vi "CUMain.vi"() -> ()   [LabVIEW 2013]
doc: "Use this template to build a simple state machine design pattern. Each state executes code and determines which state to transition to."
uses:
  controls/CUState.ctl
  controls/CUData.ctl
  <vilib>/Instr/_visa.llb/VISA Configure Serial Port (Instr).vi
panel:
  in  "Disable Encode":bool
  out "Data content":string
  out "Data length":string
  out "Package describer":string
  out "Counter":string
  in  "Send A-V command":bool
  in  "Value (U16)":u16 format="%04x"
  in  "Address (U16)":u16=255 format="%04x"
  in  "Keep send encode string":bool
  in  "Enable read":bool=TRUE
  out "Raw string":string
  in  "Bytes to read":u32=512
  out "Actual bytes read":u32
  in  "Clear text":bool
  out "Encoded string":string
  in  "Send string":string="DA1 0C1 <<< SM1 SM2 SM3 >>> MM1"
  in  "data bits":u16=8 min=5 max=8 step=1
  in  "VISA resource name":refnum<visa-resource-name>="COM1"
  in  "baud rate":u32=9600
  in  "Stop Button":bool
  in  "Send ASCII command":bool
  # "CU Console"
  # "(Add SPACE between ASCII commands)"
  # "(Press ENTER to send when value ready)"
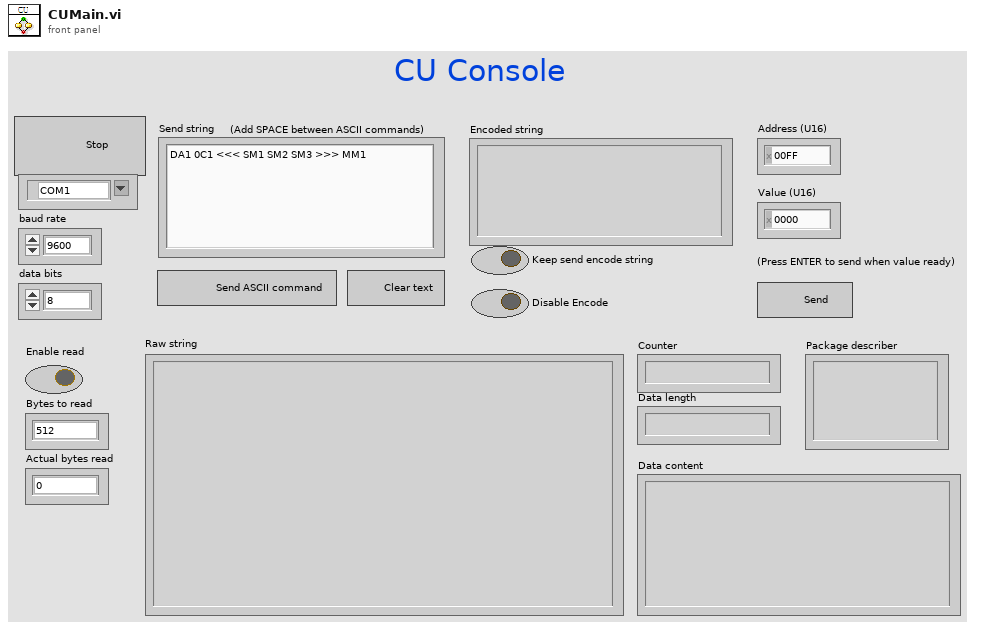
[diagram p1: front panel]
types:
  T1 = typedef "CUData.ctl" = cluster{"String to send":string, "Encoded string to send":string, "Raw string":string}
  T2 = typedef "CUState.ctl" = enum16{"Initialize", "Wait for Event", "Encode ASCII command", "Encode A-V command", "Send command", "Read data", "Decode Science data", "Stop"}
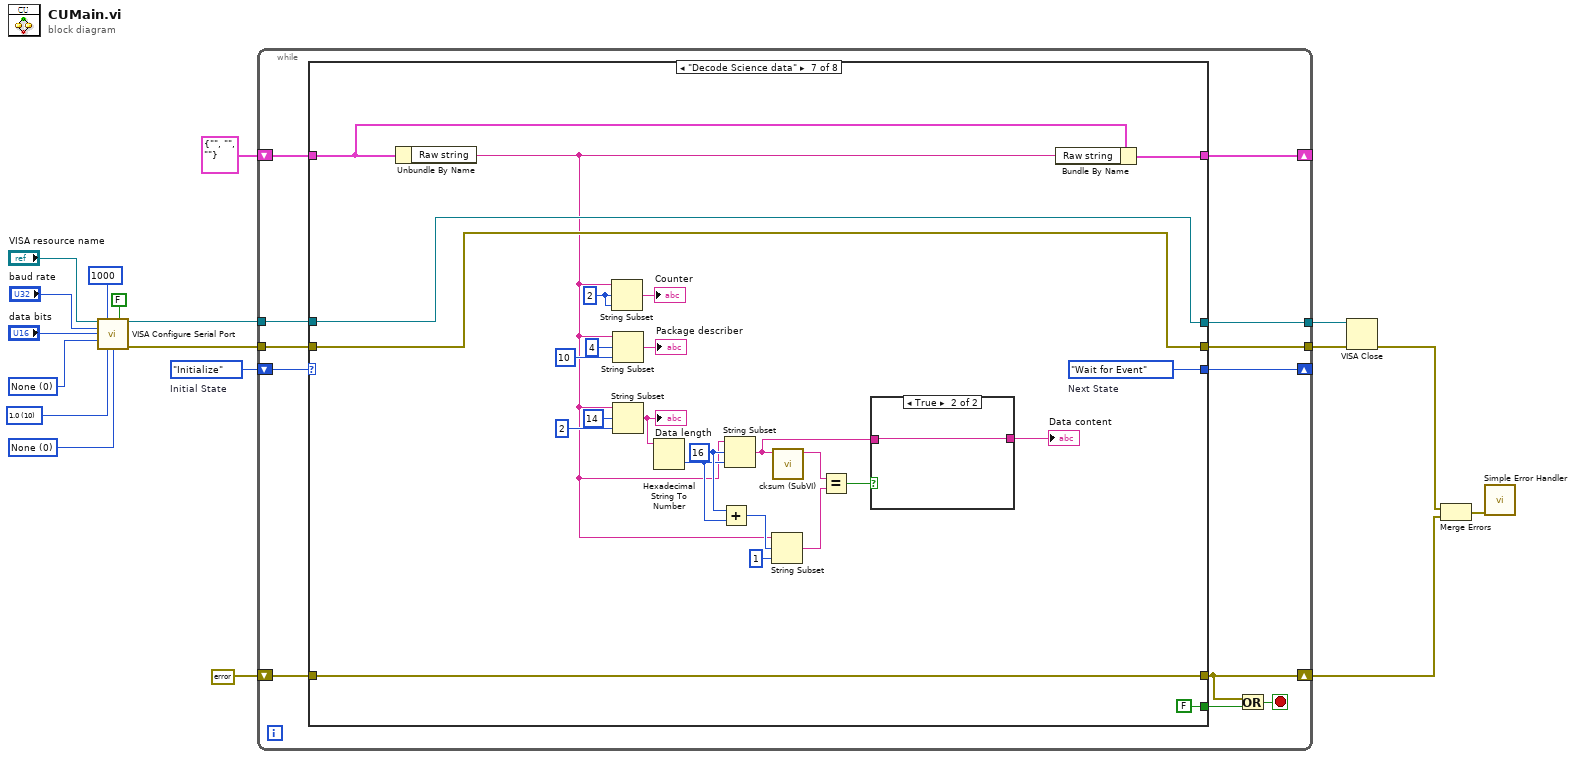
[diagram p0: block diagram]
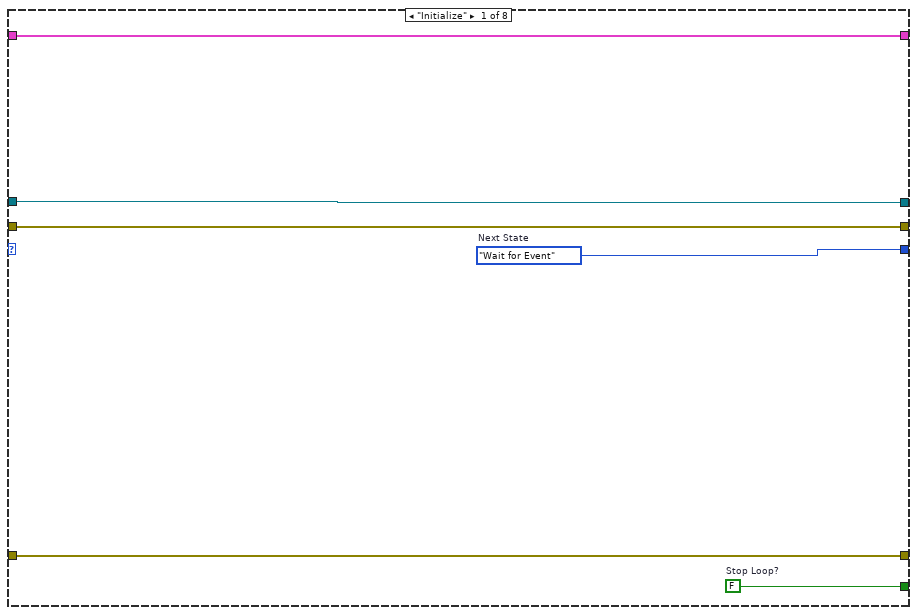
[diagram p2: hidden frame]
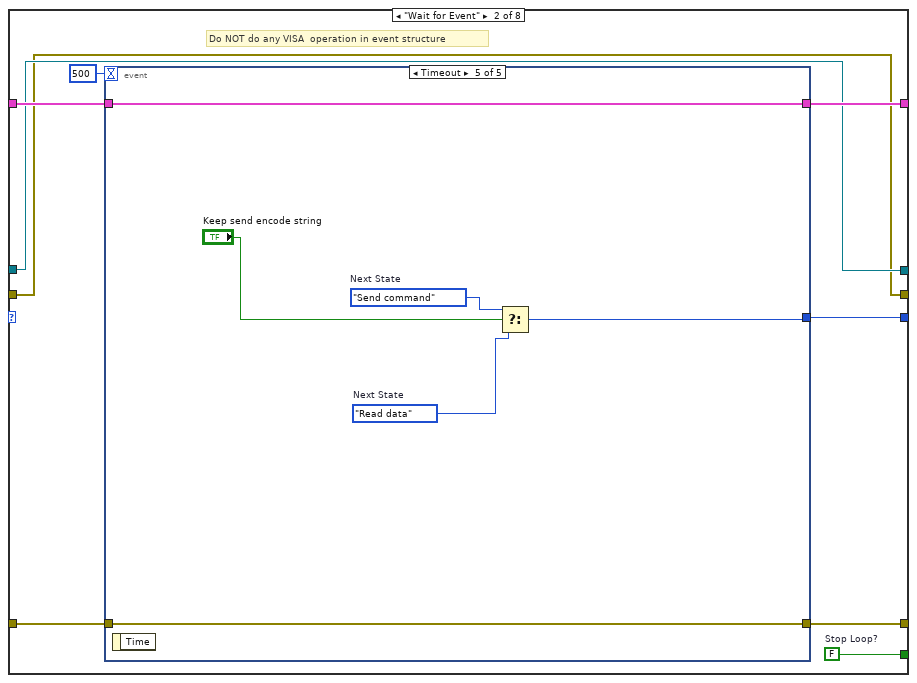
[diagram p3: hidden frame]
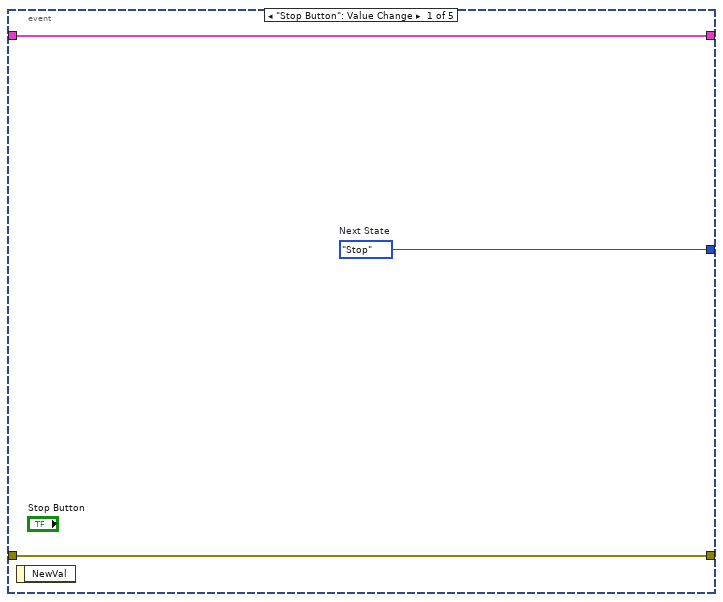
[diagram p4: hidden frame]
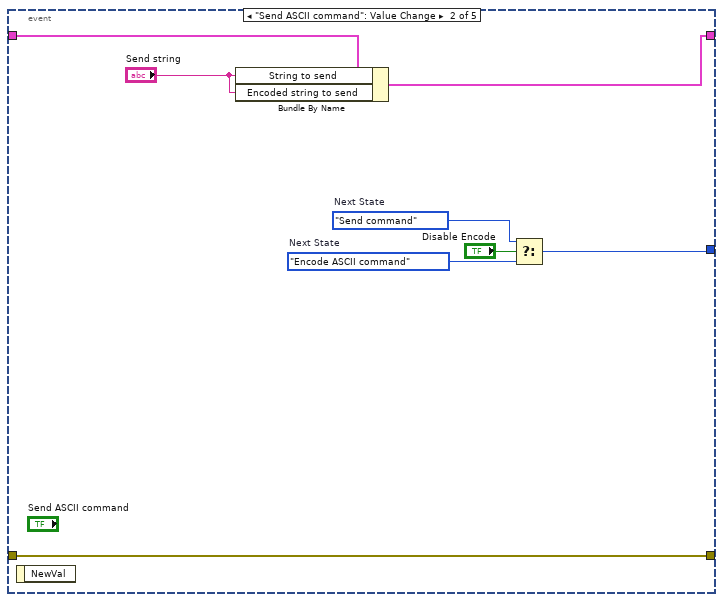
[diagram p5: hidden frame]
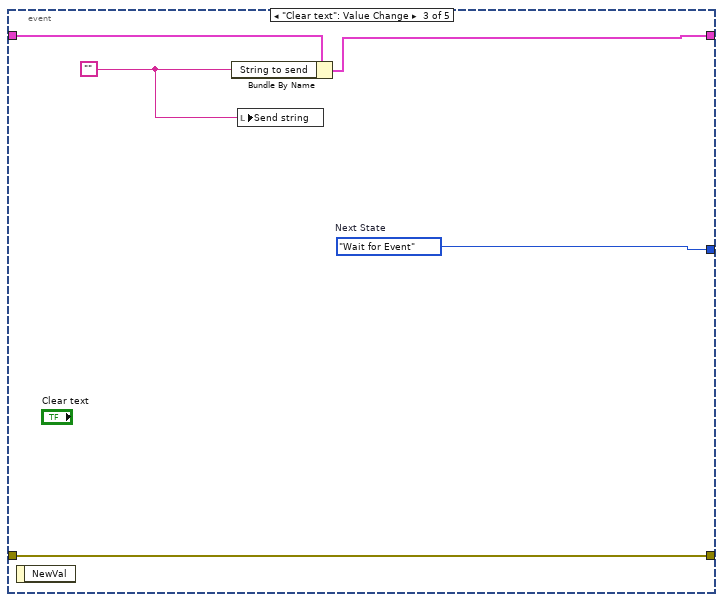
[diagram p6: hidden frame]
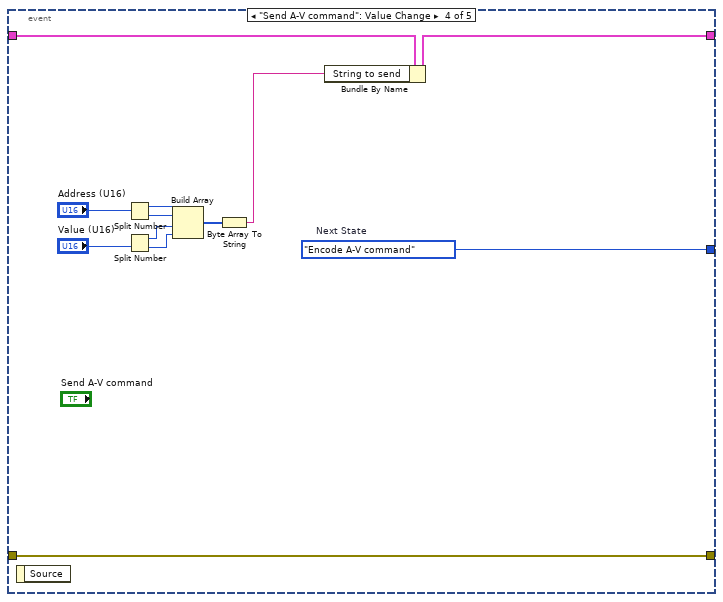
[diagram p7: hidden frame]
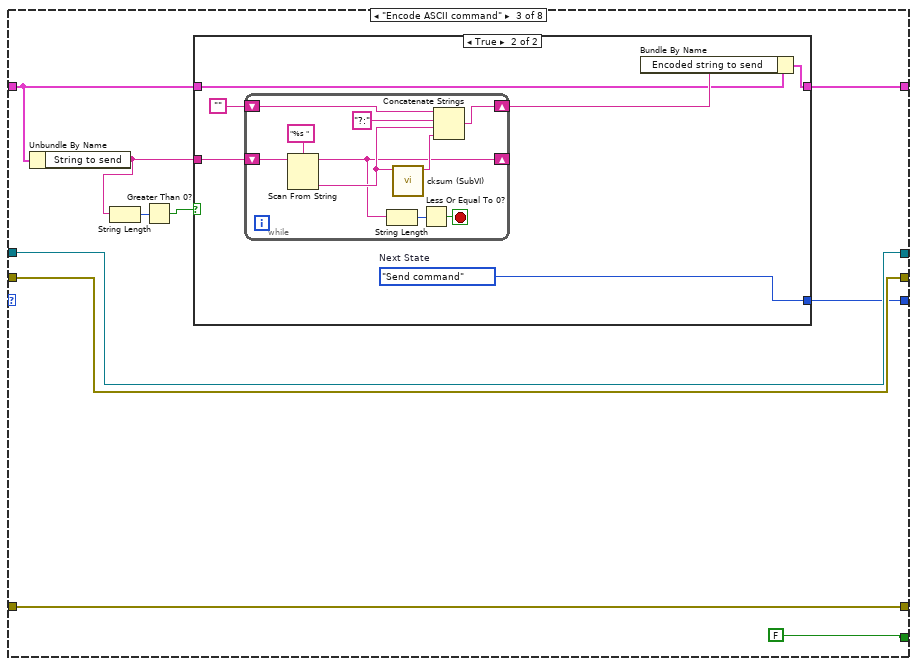
[diagram p8: hidden frame]
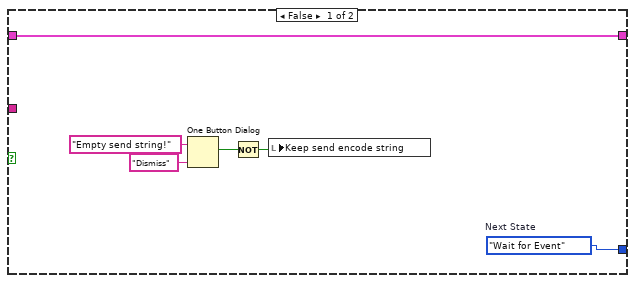
[diagram p9: hidden frame]
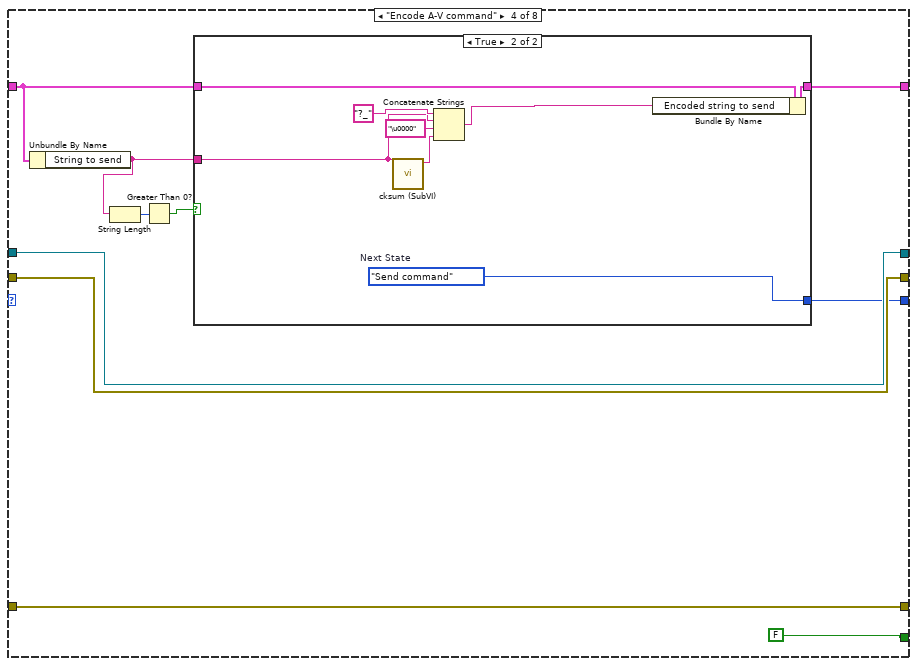
[diagram p10: hidden frame]
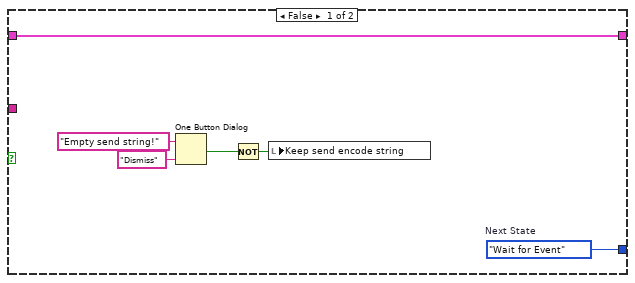
[diagram p11: hidden frame]
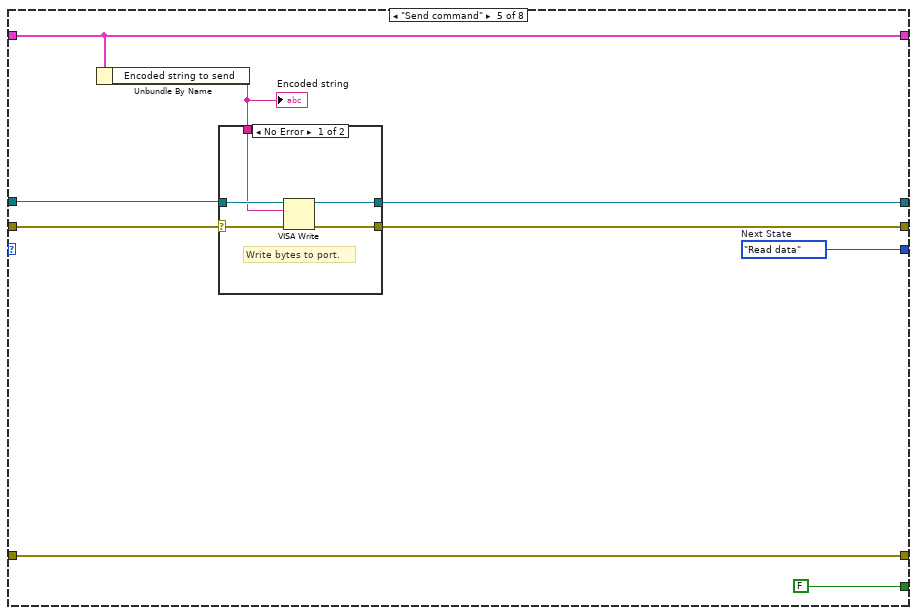
[diagram p12: hidden frame]
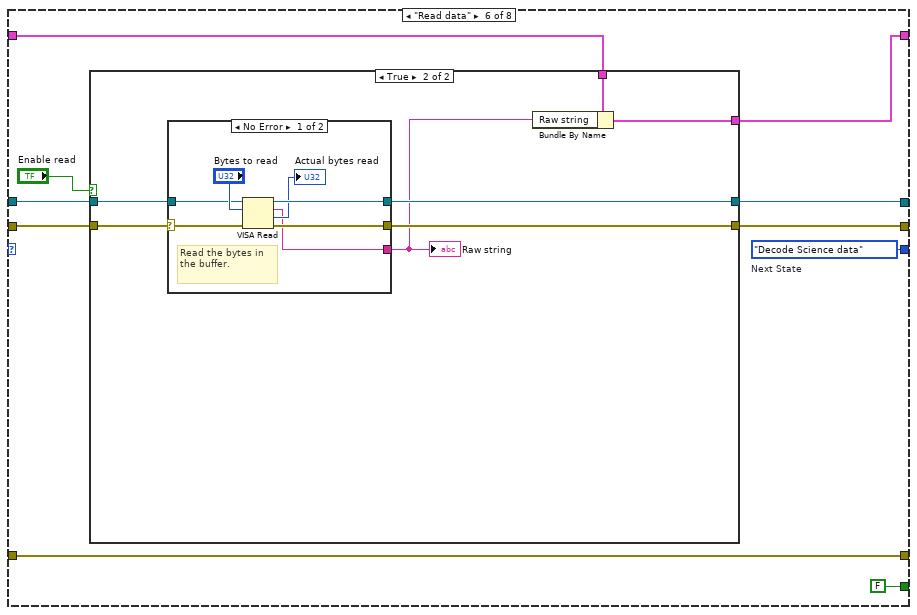
[diagram p14: hidden frame]
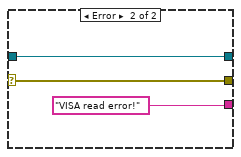
[diagram p16: hidden frame]
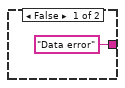
[diagram p17: hidden frame]
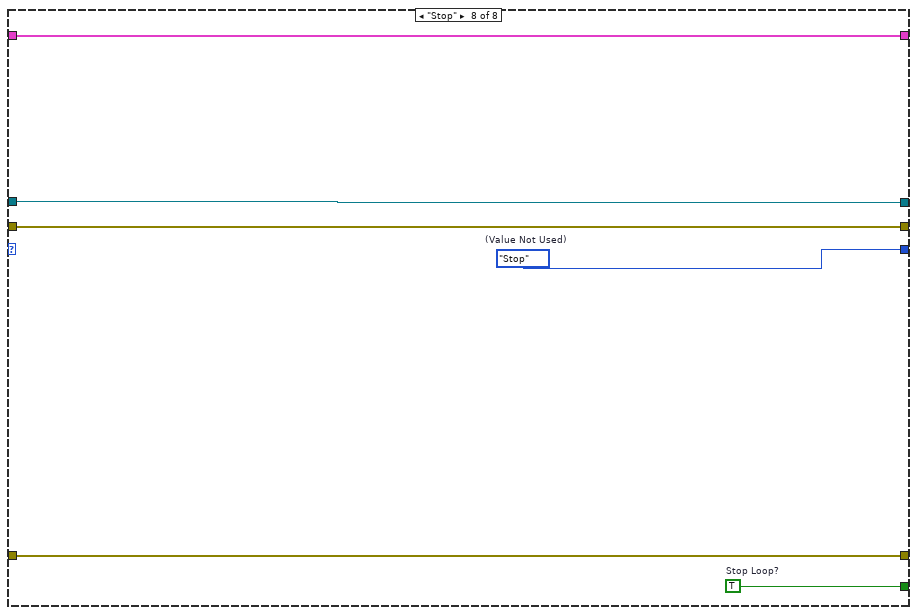
[diagram p18: hidden frame]
diagram:
  w12 = u16 10 items=["1.0"=10, "1.5"=15, "2.0"=20] ("stop bits")
  w13 = u16 0 items=["None", "Odd", "Even", "Mark", "Space"] ("parity")
  w9 = u16 0 items=["None"=0, "XON/XOFF"=1, "RTS/CTS"=2, "DTR/DSR"=4] ("flow control")
  w18 = CUState."Initialize"  # Initial State
  n1 = call-poly "VISA Configure Serial Port"("VISA resource name"="VISA resource name", "timeout (10sec)"=u32 1000 ("timeout (ms)"), "Enable Termination\nChar (T)"=FALSE ("End read on termination character?"), "baud rate (9600)"="baud rate", "data bits (8)"="data bits", "parity (0:none)"=w13, "stop bits (10: 1 bit)"=w12, "flow control (0:none)"=w9) -> ("VISA resource name out"=w6:refnum<visa-resource-name>, "error out"=w5:errorcluster)  [unwired: 2 in, 4 out]
  n2 = while {
    shift-right: [w29] -> _
    shift-left: w18 -> [w30]
    shift-right: [w27] -> _
    shift-left: T1 {"String to send"="", "Encoded string to send"="", "Raw string"=""} ("Data") -> [w28]
    shift-right: [w23] -> w1
    shift-left: errorcluster {"status"=FALSE, "code"=0, "source"=""} ("error constant") -> [w26]
    tunnel: [w22] -> w7
    tunnel: w6 -> [w21]
    tunnel: w5 -> [w20]
    tunnel: [w19] -> w4
    stop <- w24 stop-if-true
    n3 = case shown="\"Decode Science data\"" w30 {
      tunnel: [w36 w45 w86 w118 w144 w154 w187 w214] -> w29
      tunnel: [w35 w44 FALSE ("Stop Loop?") FALSE ("Stop Loop?") FALSE ("Stop Loop?") FALSE ("Stop Loop?") FALSE ("Stop Loop?") w212] -> w25
      tunnel: w28 -> [w31 w43 w84 w116 w136 w153 w184 w213]
      tunnel: [w31 w42 w83 w115 w136 w152 w185 w213] -> w27
      tunnel: w26 -> [w34 w41 w89 w121 w142 w161 w206 w211]
      tunnel: [w34 w40 w89 w121 w142 w161 w206 w211] -> w23
      tunnel: [w33 w39 w88 w120 w140 w159 w189 w210] -> w22
      tunnel: w21 -> [w33 w39 w88 w120 w141 w160 w189 w210]
      tunnel: w20 -> [w32 w38 w87 w119 w138 w157 w188 w209]
      tunnel: [w32 w38 w87 w119 w139 w158 w188 w209] -> w19
      frame "Initialize" {
        w35 = FALSE  # Stop Loop?
        w36 = CUState."Wait for Event"  # Next State
      }
      frame "Wait for Event" {
        w44 = FALSE  # Stop Loop?
        # "Do NOT do any VISA  operation in event structure"
        n4 = event shown="[4] Timeout" {
          selector: _ -> [_ _ _ _ _]
          dyn-events: _ -> [_ _ _ _ _]
          timeout: 500 -> [_ _ _ _ _]
          tunnel: [w48 w53 w58 w73 w76] -> w45
          tunnel: w43 -> [w47 w56 w60 w72 w78]
          tunnel: [w47 w55 w59 w71 w78] -> w42
          tunnel: w41 -> [w46 w54 w61 w70 w79]
          tunnel: [w46 w54 w61 w70 w79] -> w40
          event "Stop Button": Value Change {
            w48 = CUState."Stop"  # Next State
            n5 = event-data() -> ()  [unwired: 1 in, 1 out]
          }
          event "Send ASCII command": Value Change {
            w51 = CUState."Send command"  # Next State
            w52 = CUState."Encode ASCII command"  # Next State
            n6 = event-data() -> ()  [unwired: 1 in, 1 out]
            n7 = Bundle By Name(cluster=w56, "String to send"="Send string", "Encoded string to send"="Send string") -> (w55:T1)
            n8 = Select(t=w51, s="Disable Encode", f=w52) -> (s? t:f=w53:T2)
          }
          event "Clear text": Value Change {
            w58 = CUState."Wait for Event"  # Next State
            w57 = "" ("String to send")
            n9 = event-data() -> ()  [unwired: 1 in, 1 out]
            n10 = Bundle By Name(cluster=w60, "String to send"=w57) -> (w59:T1)
            n11 = local write "Send string"(w57) -> ()
          }
          event "Send A-V command": Value Change {
            w73 = CUState."Encode A-V command"  # Next State
            n12 = event-data() -> ()  [unwired: 1 in, 1 out]
            n13 = Split Number(x="Address (U16)") -> (hi(x)=w67:u8, lo(x)=w66:u8)
            n14 = Split Number(x="Value (U16)") -> (hi(x)=w65:u8, lo(x)=w64:u8)
            n15 = Build Array(w67, w66, w65, w64) -> (w63:u8[])
            n16 = Byte Array To String(unsigned byte array=w63) -> (string=w62:string)
            n17 = Bundle By Name(cluster=w72, "String to send"=w62) -> (w71:T1)
          }
          event Timeout {
            w75 = CUState."Send command"  # Next State
            w74 = CUState."Read data"  # Next State
            n18 = event-data() -> ()  [unwired: 1 in, 1 out]
            n19 = Select(t=w75, s="Keep send encode string", f=w74) -> (s? t:f=w76:T2)
          }
        }
      }
      frame "Encode ASCII command" {
        n20 = Unbundle By Name(w84) -> ("String to send"=w81:string)
        n21 = String Length(string=w81) -> (length=w82:i32)
        n22 = Greater Than 0?(x=w82) -> (x > 0?=w80:bool)
        n23 = case shown="True" w80 {
          tunnel: [w95 w101] -> w86
          tunnel: w81 -> [_ w100]
          tunnel: w84 -> [w93 w98]
          tunnel: [w93 w97] -> w83
          frame False {
            w95 = CUState."Wait for Event"  # Next State
            n24 = One Button Dialog(message="Empty send string!", button name ("OK")="Dismiss") -> (true=w90:bool)
            n25 = Not(x=w90) -> (.not. x?=w91:bool)
            n26 = local write "Keep send encode string"(w91) -> ()
          }
          frame True {
            w101 = CUState."Send command"  # Next State
            n27 = while {
              shift-right: [w104] -> _
              shift-left: w100 -> [w111]
              shift-right: [w107] -> w99
              shift-left: "" -> [w102]
              stop <- w108 stop-if-true
              n28 = Scan From String(format string="%s ", input string=w111) -> (remaining string=w104:string, output 1=w106:string)  [unwired: 3 in, 2 out]
              n29 = String Length(string=w104) -> (length=w109:i32)
              n30 = call "cksum (SubVI).vi"("Input String"=w106) -> ("Checksum"=w105:string)  [unwired: 10 in]
              n31 = Less Or Equal To 0?(x=w109) -> (x <= 0?=w108:bool)
              n32 = Concatenate Strings(w102, "?:", w106, w105) -> (w107:string)
            }
            n33 = Bundle By Name(cluster=w98, "Encoded string to send"=w99) -> (w97:T1)
          }
        }
      }
      frame "Encode A-V command" {
        n34 = Unbundle By Name(w116) -> ("String to send"=w113:string)
        n35 = String Length(string=w113) -> (length=w114:i32)
        n36 = Greater Than 0?(x=w114) -> (x > 0?=w112:bool)
        n37 = case shown="True" w112 {
          tunnel: [w127 w135] -> w118
          tunnel: w113 -> [_ w129]
          tunnel: w116 -> [w125 w133]
          tunnel: [w125 w132] -> w115
          frame False {
            w127 = CUState."Wait for Event"  # Next State
            n38 = One Button Dialog(message="Empty send string!", button name ("OK")="Dismiss") -> (true=w122:bool)
            n39 = Not(x=w122) -> (.not. x?=w123:bool)
            n40 = local write "Keep send encode string"(w123) -> ()
          }
          frame True {
            w135 = CUState."Send command"  # Next State
            n41 = call "cksum (SubVI).vi"("Input String"=w129) -> ("Checksum"=w131:string)  [unwired: 10 in]
            n42 = Concatenate Strings("?_", w129, "\u0000" ("string"), w131) -> (w134:string)
            n43 = Bundle By Name(cluster=w133, "Encoded string to send"=w134) -> (w132:T1)
          }
        }
      }
      frame "Send command" {
        w144 = CUState."Read data"  # Next State
        n44 = Unbundle By Name(w136) -> ("Encoded string to send"=w137:string)
        "Encoded string" <- w137
        n45 = case shown="No Error" w138 {
          selector: w138 -> [w146 w151]
          tunnel: [w149 w150] -> w140
          tunnel: [w148 w151] -> w139
          tunnel: w141 -> [w147 w150]
          tunnel: w137 -> [w145 _]
          frame No Error {
            # "Write bytes to port."
            n46 = VISA Write(VISA resource name=w147, write buffer=w145, error in (no error)=w146) -> (VISA resource name out=w149:refnum<visa-resource-name>, error out=w148:errorcluster)  [unwired: 1 out]
          }
          frame Error {
          }
        }
      }
      frame "Read data" {
        w154 = CUState."Decode Science data"  # Next State
        n47 = case shown="True" "Enable read" {
          tunnel: w160 -> [w164 w171]
          tunnel: [w164 w170] -> w159
          tunnel: [w163 w169] -> w158
          tunnel: w157 -> [w163 w168]
          tunnel: w153 -> [w162 w167]
          tunnel: [w162 w165] -> w152
          frame False {
          }
          frame True {
            n48 = case "Read bytes from port." shown="No Error" w168 {
              selector: w168 -> [w174 w180]
              tunnel: [w177 w180] -> w169
              tunnel: [w178 w181] -> w170
              tunnel: w171 -> [w175 w181]
              tunnel: [w172 "VISA read error!" ("read buffer")] -> w166
              frame No Error {
                # "Read the bytes in the buffer."
                n49 = VISA Read(VISA resource name=w175, byte count="Bytes to read", error in (no error)=w174) -> (VISA resource name out=w178:refnum<visa-resource-name>, read buffer=w172:string, return count=→"Actual bytes read":u32, error out=w177:errorcluster)
              }
              frame Error {
                # "Error occurred \nreading Bytes at \nSerial Port"
              }
            }
            "Raw string" <- w166
            n50 = Bundle By Name(cluster=w167, "Raw string"=w166) -> (w165:T1)
          }
        }
      }
      frame "Decode Science data" {
        w187 = CUState."Wait for Event"  # Next State
        w197 = u32 16 ("offset (0)")
        w198 = 2 ("offset (0)")
        n51 = Unbundle By Name(w184) -> ("Raw string"=w183:string)
        n52 = String Subset(string=w183, offset (0)=w198, length (rest)=w198) -> (substring=→"Counter":string)
        n53 = String Subset(string=w183, offset (0)=4, length (rest)=10 ("length (rest)")) -> (substring=→"Package describer":string)
        n54 = String Subset(string=w183, offset (0)=14, length (rest)=2 ("length (rest)")) -> (substring=w200:string)
        "Data length" <- w200
        n55 = Hexadecimal String To Number(string=w200) -> (number=w196:u32)  [unwired: 2 in, 1 out]
        n56 = Add(x=w197, y=w196) -> (x+y=w195:u32)
        n57 = String Subset(string=w183, offset (0)=w197, length (rest)=w196) -> (substring=w190:string)
        n58 = String Subset(string=w183, offset (0)=w195, length (rest)=1 ("length (rest)")) -> (substring=w192:string)
        n59 = call "cksum (SubVI).vi"("Input String"=w190) -> ("Checksum"=w193:string)  [unwired: 10 in]
        n60 = Equal?(x=w193, y=w192) -> (x = y?=w191:bool)
        n61 = case shown="True" w191 {
          tunnel: w190 -> [_ w208]
          tunnel: ["Data error" ("Raw string") w208] -> w182
          frame False {
          }
          frame True {
          }
        }
        "Data content" <- w182
        n62 = Bundle By Name(cluster=w184, "Raw string"=w183) -> (w185:T1)
      }
      frame "Stop" {
        w212 = TRUE  # Stop Loop?
        w214 = CUState."Stop"  # (Value Not Used)
      }
    }
    n63 = Or(x=w23, y=w25) -> (x .or. y?=w24:bool)
  }
  n64 = VISA Close(VISA resource name=w7, error in (no error)=w4) -> (error out=w2:errorcluster)
  n65 = Merge Errors(w2, w1) -> (w3:errorcluster)
  n66 = call <vilib>:"Simple Error Handler.vi"("error in (no error)"=w3) -> ()  [unwired: 4 in, 5 out]
